vi "RT Loop - Data Acquisition.vi"(8 "error in (no error)":errorcluster caption="错误输入（无错误）", 11 "Message Queues":T1 caption="消息队列") -> (0 "error out":errorcluster caption="错误输出")   [LabVIEW 2015]
uses:
  Message Queue/All Real-Time Message Queues.ctl
  Message Queue/Message Cluster.ctl
  Globals/Global - Monitoring Variables.vi
  Message Queue/Message Queue.lvlib
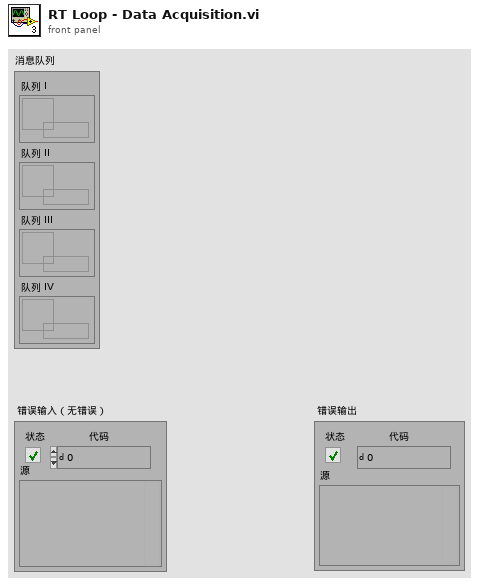
[diagram p1: front panel]
types:
  T1 = typedef "Message Queue.lvlib/All Real-Time Message Queues.ctl" = cluster{"Queue I":refnum<queue>, "Queue II":refnum<queue>, "Queue III":refnum<queue>, "Queue IV":refnum<queue>}
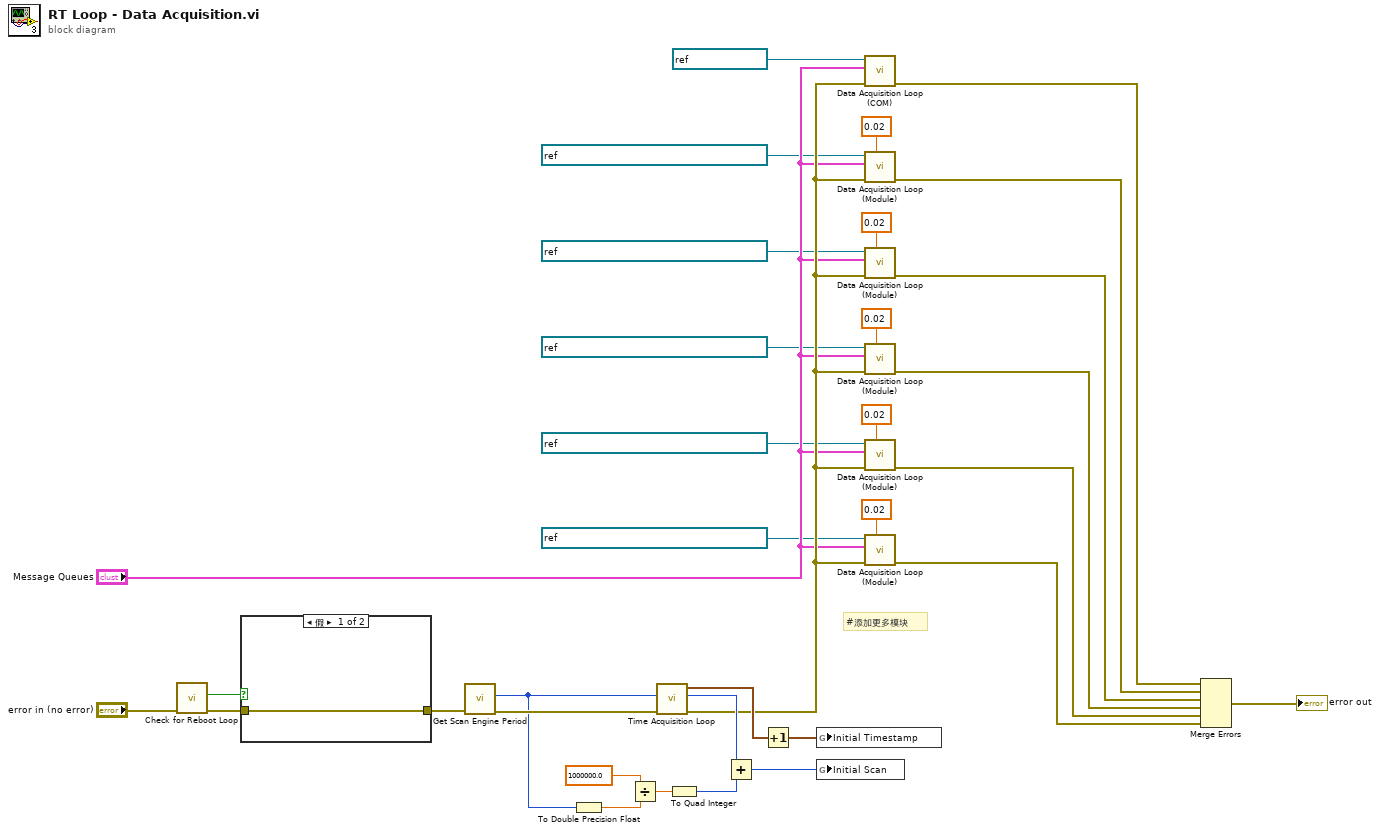
[diagram p0: block diagram]
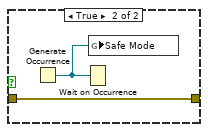
[diagram p2: hidden frame]
diagram:
  # "#添加更多模块"
  n1 = call "Check for Reboot Loop.vi"("error in (no error)"="error in (no error)") -> ("error out"=w19:errorcluster, "Start in Safe Mode?"=w20:bool)  [unwired: 9 in]
  n2 = case shown="假" w20 {
    tunnel: w19 -> [w35 w37]
    tunnel: [w35 w37] -> w18
    frame False {
    }
    frame True {
      n3 = Generate Occurrence() -> (w36:refnum<k4>)
      n4 = Wait on Occurrence(2:w36) -> ()  [unwired: 2 in, 1 out]
      n5 = global write "Global - Monitoring Variables.vi" "Safe Mode"(w36) -> ()
    }
  }
  n6 = call <vilib>:"Get Scan Engine Period.vi"("error in (no error)"=w18) -> ("scan period (uSec)"=w22:u32, "error out"=w25:errorcluster)  [unwired: 13 in]
  n7 = To Double Precision Float(number=w22) -> (double precision float=w27:dbl)
  n8 = Divide(x=1000000.0, y=w27) -> (x/y=w28:dbl)
  n9 = call "Time Acquisition Loop.vi"("error in (no error)"=w25, "scan period (uSec)"=w22) -> ("error out"=w13:errorcluster, "Scan Engine Time"=w29:i64, "Timestamp"=w31:timestamp)  [unwired: 7 in]
  n10 = To Quad Integer(1:w28) -> (0:w26:i64)
  n11 = Add(x=w29, y=w26) -> (x+y=w23:i64)
  n12 = Increment(x=w31) -> (x+1=w24:timestamp)
  n13 = global write "Global - Monitoring Variables.vi" "Initial Timestamp"(w24) -> ()
  n14 = global write "Global - Monitoring Variables.vi" "Initial Scan"(w23) -> ()
  n15 = call "Data Acquisition Loop (COM).vi"("error in (no error)"=w13, "Message Queues"="Message Queues", "VISA resource name"=refnum<visa-resource-name> "USB2RS485") -> ("error out"=w14:errorcluster)  [unwired: 8 in]
  n16 = call "Data Acquisition Loop (Module).vi"("Sampling Period (S)"=0.02 ("Sampling Period(S)"), "error in (no error)"=w13, "Message Queues"="Message Queues", "IO Container"=refnum<k21> "ni.var.io://ni-crio-9036-dxlq/Mod8" ("9219 Refnum")) -> ("error out"=w15:errorcluster)  [unwired: 7 in]
  n17 = call "Data Acquisition Loop (Module).vi"("Sampling Period (S)"=0.02 ("Sampling Period(S)"), "error in (no error)"=w13, "Message Queues"="Message Queues", "IO Container"=refnum<k21> "ni.var.io://ni-crio-9036-dxlq/Mod6" ("9219 Refnum")) -> ("error out"=w16:errorcluster)  [unwired: 7 in]
  n18 = call "Data Acquisition Loop (Module).vi"("Sampling Period (S)"=0.02 ("Sampling Period(S)"), "error in (no error)"=w13, "Message Queues"="Message Queues", "IO Container"=refnum<k21> "ni.var.io://ni-crio-9036-dxlq/Mod4" ("9219 Refnum")) -> ("error out"=w33:errorcluster)  [unwired: 7 in]
  n19 = call "Data Acquisition Loop (Module).vi"("Sampling Period (S)"=0.02 ("Sampling Period(S)"), "error in (no error)"=w13, "Message Queues"="Message Queues", "IO Container"=refnum<k21> "ni.var.io://ni-crio-9036-dxlq/Mod2" ("9219 Refnum")) -> ("error out"=w32:errorcluster)  [unwired: 7 in]
  n20 = call "Data Acquisition Loop (Module).vi"("Sampling Period (S)"=0.02 ("Sampling Period(S)"), "error in (no error)"=w13, "Message Queues"="Message Queues", "IO Container"=refnum<k21> "ni.var.io://ni-crio-9036-dxlq/Mod1" ("9239 Refnum")) -> ("error out"=w17:errorcluster)  [unwired: 7 in]
  n21 = Merge Errors(w14, w15, w16, w33, w32, w17) -> (→"error out":errorcluster)
